vi "Stop Core.vi"(10 "final error code":i32, 11 "Series Actor in":refnum<class "Series Actor.lvclass">) -> (3 "Series Actor out":refnum<class "Series Actor.lvclass">)   [LabVIEW 2023, in "Series Actor.lvlib" / "Series Actor.lvclass"]
doc: "(<B>Filename</B>: Actor Framework.lvlib:Actor.lvclass:Stop Core.vi)\n\nDefines what the actor does before it stops. Use the <B>final error code</B> input to determine whether the actor shut down in response to an error.\n\nBy default, this method passes the Stop message along to all auto-stop nested actors. A descendant class may override this method to define additional behavior, such as shutting down any processes the actor initiated in its override of the Actor Core method."
uses:
  Series Actor.lvclass
  Series Actor.lvclass/Series Actor.ctl
  <vilib>/MGI/Panel Manager/Panel Actor/Panel Actor/Panel Actor.lvclass
  HAL/MSS/MSS.lvclass
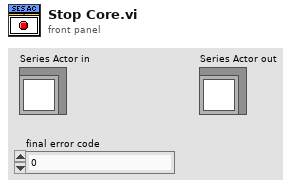
[diagram p1: front panel]
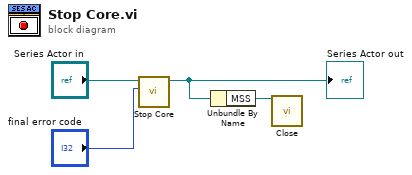
[diagram p0: block diagram]
diagram:
  n1 = call-parent "Stop Core.vi"("final error code"="final error code", "Actor in"="Series Actor in") -> ("Actor out"=w2:refnum<class "Series Actor.lvclass">)  [unwired: 9 in]
  "Series Actor out" <- w2
  n2 = Unbundle By Name(w2) -> ("MSS"=w1:refnum<class "MSS.lvclass">)
  n3 = call "Close.vi"("MSS in"=w1) -> ()  [unwired: 9 in, 2 out]
